vi "Goal Vision Align.vi"(6 "Reinitialize?":bool, 7 "PID gains":T1={"proportional gain (Kc)"=1.0, "integral time (Ti, min)"=0.01, "derivative time (Td, min)"=0.0} {"derivative time (Td, min)" format="%.3f"; "integral time (Ti, min)" format="%.3f"; "proportional gain (Kc)" format="%.3f"}, 8 "Gyro Tolerance":dbl, 9 "X Min":dbl, 10 "X Max":dbl, 11 "Goal Angle Difference":dbl) -> (0 "Finished?":bool, 1 "Heading Target":dbl, 3 "X Out":dbl)   [LabVIEW 2016]
uses:
  Common Code/PID Gains.ctl
  Robot Global Data.vi
  <vilib>/addons/control/pid/pid.llb/PID (DBL).vi
  <vilib>/addons/control/pid/NI_PID_pid.lvlib
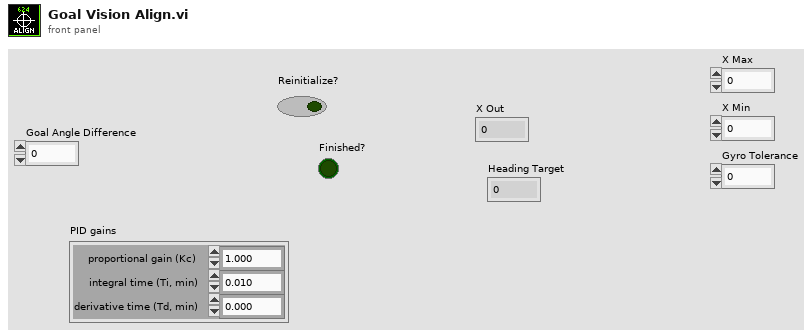
[diagram p1: front panel]
types:
  T1 = typedef "PID Gains.ctl" = cluster{"proportional gain (Kc)":dbl, "integral time (Ti, min)":dbl, "derivative time (Td, min)":dbl}
  T2 = typedef "Drivetrain Status Cluster.ctl" = cluster{"Drivetrain Mode":enum16{"Manual", "Gyro Steer"}, "Y (Throttle)":dbl, "X (Steer)":dbl, "Z (Strafe)":dbl, "Heading Target":dbl, "Center Piston Down?":bool, "Traction?":bool, "Gyro Steer Finished?":bool, "Distance Drive Finished?":bool, "Gyro":dbl, "Distance Target":dbl, "Y Max Output":dbl, "Y Min Output":dbl, "X Max Output":dbl, "X Min Output":dbl, "Z Max Output":dbl, "Z Min Output":dbl, "Translation Target":dbl, "Translation Drive Finished?":bool, "PID Auto Drive Finished?":bool, "Brake?":bool, "Vision Aligned?":bool, "Creep Mode Engaged?":bool}
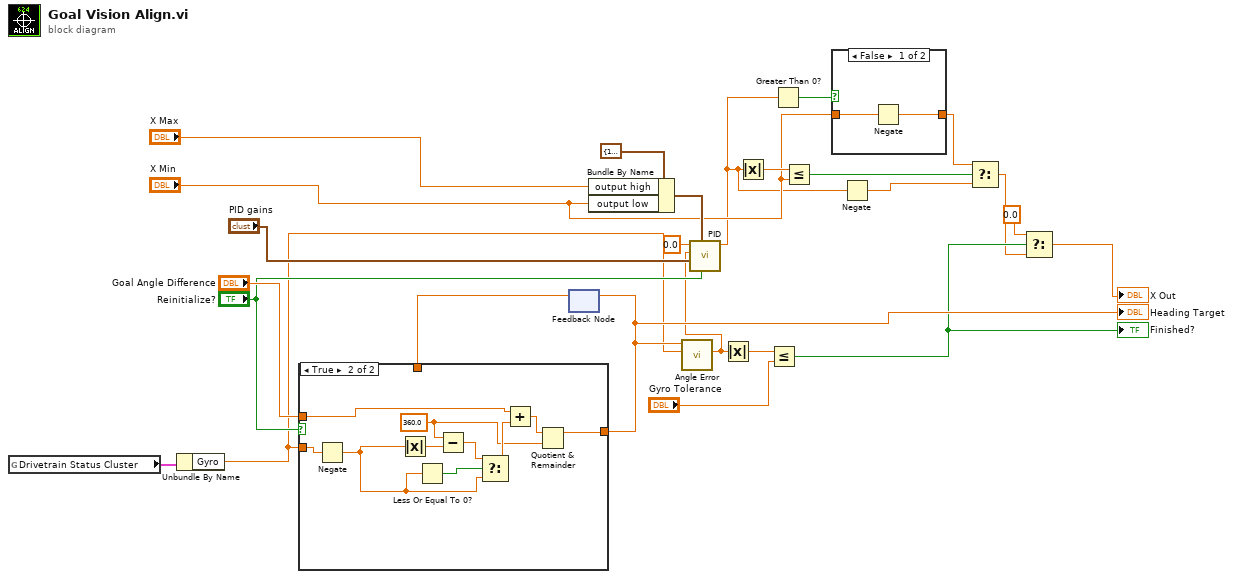
[diagram p0: block diagram]
diagram:
  n1 = global read "Robot Global Data.vi" "Drivetrain Status Cluster"() -> (w4:T2)
  n2 = Unbundle By Name(w4) -> ("Gyro"=w3:dbl)
  n3 = feedback #1() -> (w24:dbl)  [unwired: 1 in]
  n4 = case shown="True" "Reinitialize?" {
    tunnel: [w26 w27] -> w12
    tunnel: "Goal Angle Difference" -> [_ w30]
    tunnel: w3 -> [_ w32]
    tunnel: w24 -> [w26 _]
    frame False {
    }
    frame True {
      w28 = 360.0 ("x")
      n5 = Negate(x=w32) -> (-x=w33:dbl)
      n6 = Absolute Value(x=w33) -> (abs(x)=w35:dbl)
      n7 = Less Or Equal To 0?(x=w33) -> (x <= 0?=w36:bool)
      n8 = Subtract(x=w28, y=w35) -> (x-y=w34:dbl)
      n9 = Select(t=w34, s=w36, f=w33) -> (s? t:f=w31:dbl)
      n10 = Add(x=w30, y=w31) -> (x+y=w29:dbl)
      n11 = Quotient & Remainder(x=w29, y=w28) -> (x-y*floor(x/y)=w27:dbl)  [unwired: 1 out]
    }
  }
  "Heading Target" <- w12
  n12 = feedback-in #1(w12) -> ()
  n13 = Bundle By Name(cluster=cluster{"output high":dbl, "output low":dbl} {"output high"=100.0, "output low"=-100.0} ("output range"), "output high"="X Max", "output low"="X Min") -> (w20:cluster{"output high":dbl, "output low":dbl})
  n14 = call "Angle Error.vi"("Angle"=w3, "Target Angle"=w12) -> ("Error"=w1:dbl)  [unwired: 9 in]
  n15 = call-poly <vilib>:"PID.vi"("reinitialize? (F)"="Reinitialize?", "output range"=w20, "PID gains"="PID gains", "process variable"=w1, "setpoint"=0.0) -> ("output"=w13:dbl)  [unwired: 5 in, 1 out]
  n16 = Absolute Value(x=w1) -> (abs(x)=w11:dbl)
  n17 = Absolute Value(x=w13) -> (abs(x)=w17:dbl)
  n18 = Less Or Equal?(x=w11, y="Gyro Tolerance") -> (x <= y?=w9:bool)
  "Finished?" <- w9
  n19 = Greater Than 0?(x=w13) -> (x > 0?=w18:bool)
  n20 = Less Or Equal?(x=w17, y="X Min") -> (x <= y?=w15:bool)
  n21 = case shown="False" w18 {
    tunnel: "X Min" -> [w38 w39]
    tunnel: [w37 w39] -> w14
    frame False {
      n22 = Negate(x=w38) -> (-x=w37:dbl)
    }
    frame True {
    }
  }
  n23 = Negate(x=w13) -> (-x=w5:dbl)
  n24 = Select(t=w14, s=w15, f=w5) -> (s? t:f=w8:dbl)
  n25 = Select(t=0.0, s=w9, f=w8) -> (s? t:f=→"X Out":dbl)
